vi "Create.vi"(6 "Year of license":i32, 8 "error in (no error)":errorcluster, 10 "Company_Info":T1, 11 "Object License Manager in":refnum<class "Software License Manager.lvclass">) -> (0 "error out":errorcluster, 1 "ok?":bool, 3 "Object License Manager out":refnum<class "Software License Manager.lvclass">)   [LabVIEW 2025, in "SW License Manager.lvlib" / "Software License Manager.lvclass"]
uses:
  Software License Manager.lvclass
  CompanyInfo--cluster.ctl
  Software License Manager.lvclass/Software License Manager.ctl
  Board/Board.lvclass/Board.ctl
  Properties/Read Website.vi
  Properties/Read Secret Key for License Verification Requests.vi
  Properties/Read Product_Ref.vi
  Properties/Read Board.vi
  Board/Read Product ID.vi
  <vilib>/httpClient/POSTBuffer.vi
  Board/Board.lvclass
  <vilib>/httpClient/LabVIEWHTTPClient.lvlib
  SW License Manager.lvlib
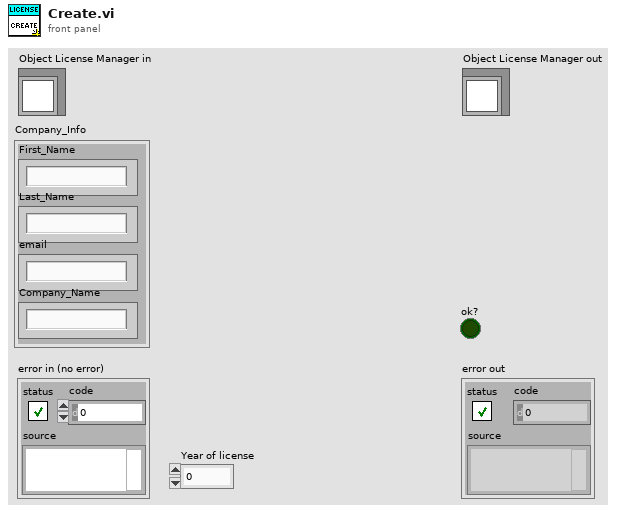
[diagram p1: front panel]
types:
  T1 = typedef "SW License Manager.lvlib/CompanyInfo--cluster.ctl" = cluster{"First_Name":string, "Last_Name":string, "email":string, "Company_Name":string}
  T2 = typedef "LVDateTimeRec.ctl" = cluster{"fractional second":dbl, "second":i32, "minute":i32, "hour":i32, "day of month":i32, "month":i32, "year":i32, "day of week":i32, "day of year":i32, "DST":i32}
  T3 = typedef "LabVIEWHTTPClient.lvlib/ClientHandle.ctl" = refnum<k1>
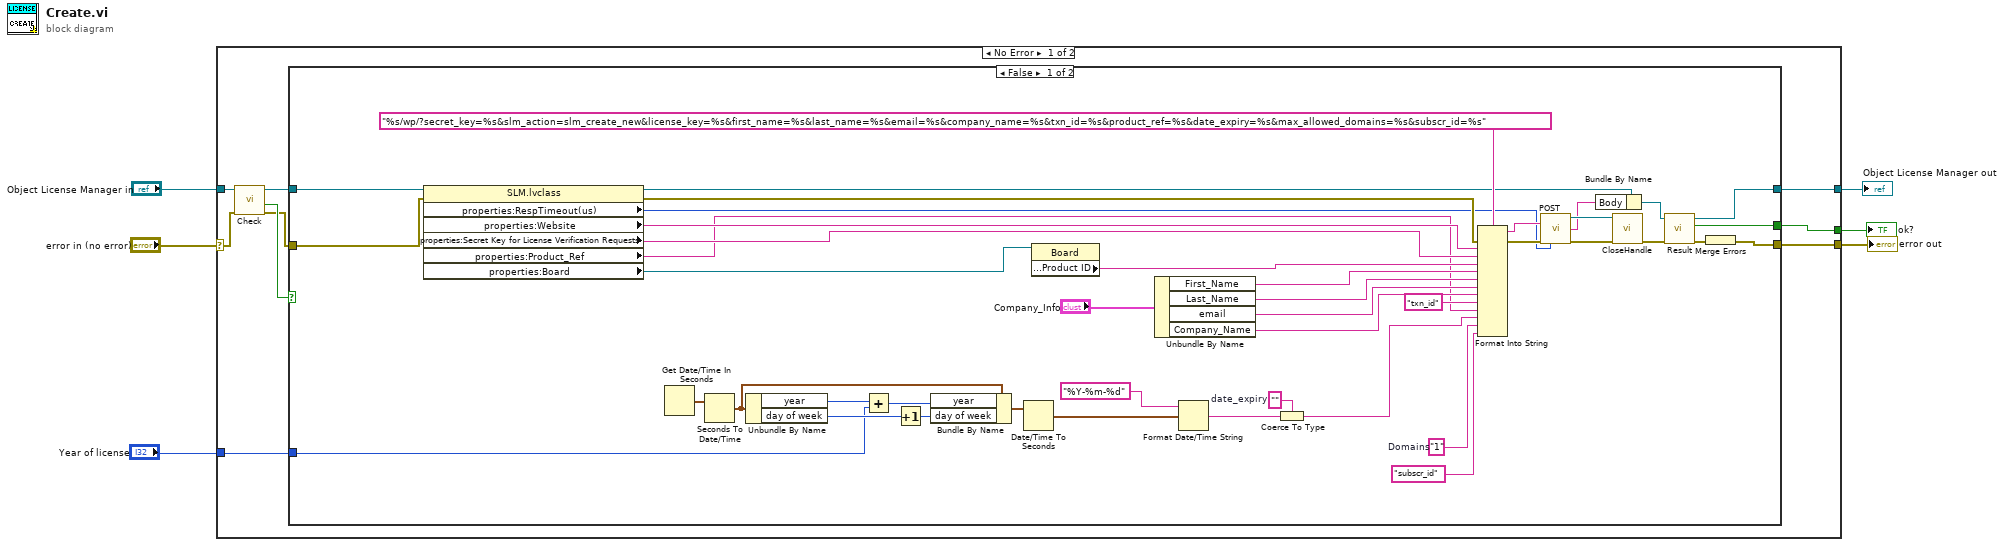
[diagram p0: block diagram]
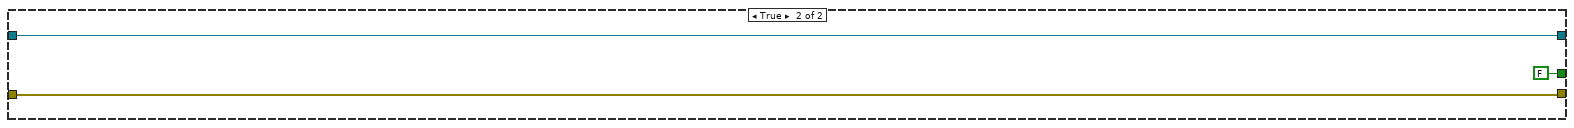
[diagram p2: hidden frame]
diagram:
  n1 = case shown="No Error" "error in (no error)" {
    selector: "error in (no error)" -> [w8 w63]
    tunnel: [w15 w63] -> w5
    tunnel: [w14 w62] -> w3
    tunnel: "Object License Manager in" -> [w12 w62]
    tunnel: [w13 _] -> w2
    tunnel: "Year of license" -> [w10 _]
    frame No Error {
      n2 = call-dynamic "Check.vi"("error in (no error)"=w8, "Object License Manager in"=w12) -> ("error out"=w7:errorcluster, "ok?"=w11:bool, "Object License Manager out"=w9:refnum<class "Software License Manager.lvclass">)  [unwired: 6 in, 1 out]
      n3 = case shown="False" w11 {
        tunnel: w7 -> [w20 w61]
        tunnel: [w47 w61] -> w15
        tunnel: [w43 w60] -> w14
        tunnel: [w42 FALSE ("ok?")] -> w13
        tunnel: w9 -> [w24 w60]
        tunnel: w10 -> [w25 _]
        frame False {
          w39 = ""  # date_expiry
          w30 = "1"  # Domains
          n4 = property class="SLM.lvclass"(reference=w24, error in=w20) -> (reference out=w21:refnum<class "Software License Manager.lvclass">, error out=w19:errorcluster, "properties:RespTimeout(us)"=w16:i32, "properties:Website"=w23:string, "properties:Secret Key for License Verification Requests"=w22:string, "properties:Product_Ref"=w18:string, "properties:Board"=w17:refnum<class "Board.lvclass">)
          n5 = Get Date/Time In Seconds() -> (seconds since 1Jan1904=w32:timestamp)
          n6 = Seconds To Date/Time(time stamp (now)=w32) -> (date time rec=w35:T2)  [unwired: 1 in]
          n7 = Unbundle By Name(w35) -> ("year"=w27:i32, "day of week"=w33:i32)
          n8 = Add(x=w27, y=w25) -> (x+y=w26:i32)
          n9 = Increment(x=w33) -> (x+1=w34:i32)
          n10 = Bundle By Name(cluster=w35, "year"=w26, "day of week"=w34) -> (w36:T2)
          n11 = Date/Time To Seconds(2:w36) -> (0:w37:timestamp)  [unwired: 1 in]
          n12 = property class="Board"(reference=w17) -> ("properties:Product ID"=w28:string)  [unwired: 1 in, 2 out]
          n13 = Unbundle By Name("Company_Info") -> ("First_Name"=w56:string, "Last_Name"=w55:string, "email"=w54:string, "Company_Name"=w53:string)
          n14 = Format Date/Time String(time format string (%c)="%Y-%m-%d", seconds (now)=w37) -> (date/time string=w38:string)  [unwired: 1 in]
          n15 = Coerce To Type(0:w38, 1:w39) -> (2:w31:string)
          n16 = Format Into String(format string="%s/wp/?secret_key=%s&slm_action=slm_create_new&license_key=%s&first_name=%s&last_name=%s&email=%s&company_name=%s&txn_id=%s&product_ref=%s&date_expiry=%s&max_allowed_domains=%s&subscr_id=%s", error in=w19, w23, w22, w28, w56, w55, w54, w53, "txn_id", w18, w31, w30, "subscr_id") -> (resulting string=w52:string, error out=w51:errorcluster)  [unwired: 1 in]
          n17 = call-poly <vilib>:"POST.vi"("url"=w52, "error in (no error)"=w51, "timeout (10000)"=w16) -> ("client handle out"=w49:T3, "body"=w45:string, "error out"=w50:errorcluster)  [unwired: 9 in, 1 out]
          n18 = Bundle By Name(cluster=w21, "Body"=w45) -> (w44:refnum<class "Software License Manager.lvclass">)
          n19 = call <vilib>:"CloseHandle.vi"("client handle"=w49, "error in (no error)"=w50) -> ("error out"=w48:errorcluster)  [unwired: 13 in]
          n20 = call-dynamic "Result.vi"("error in (no error)"=w48, "Software License Manager in"=w44) -> ("error out"=w46:errorcluster, "ok?"=w42:bool, "Software License Manager out"=w43:refnum<class "Software License Manager.lvclass">)  [unwired: 6 in, 1 out]
          n21 = Merge Errors(w46) -> (w47:errorcluster)
        }
        frame True {
        }
      }
    }
    frame Error {
    }
  }
  "error out" <- w5
  "Object License Manager out" <- w3
  "ok?" <- w2
